vi "电流特性判定.vi"(7 "Result":refnum<vi>, 9 "索引":u8, 10 "判定参数":T1, 11 "XY曲线":cluster{"X":dbl[], "Y":dbl[]}[](array[cluster])) -> (2 "判定项长度":i32, 3 "OK？":bool)   [LabVIEW 2020]
panel:
  out "对称性检测点":dbl
  out "目标5逆向输入扭矩":dbl
  out "目标5正向输入扭矩":dbl
  out "目标 5":dbl
  out "目标4逆向输入扭矩":dbl
  out "目标4正向输入扭矩":dbl
  out "目标 4":dbl
  out "目标3逆向输入扭矩":dbl
  out "目标3正向输入扭矩":dbl
  out "目标 3":dbl
  out "目标2逆向输入扭矩":dbl
  out "目标2正向输入扭矩":dbl
  out "目标 2":dbl
  out "目标1正向输入扭矩":dbl
  out "目标1逆向输入扭矩":dbl
  out "目标 1":dbl
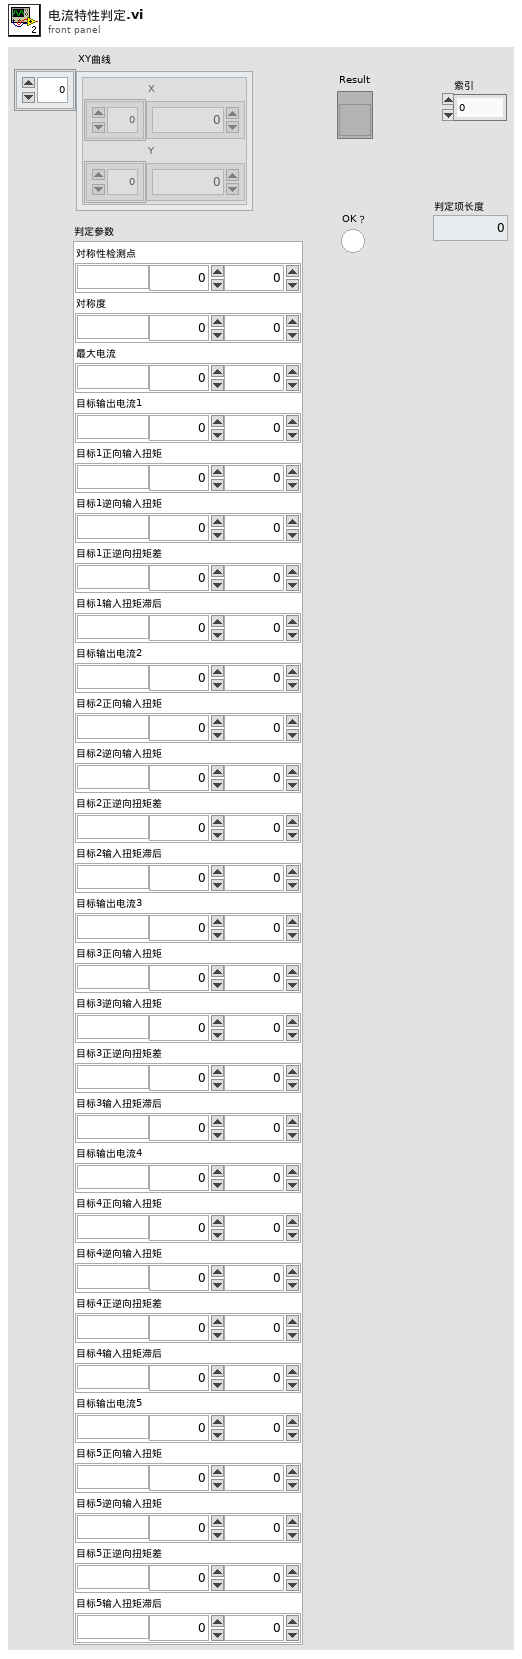
[diagram p1: front panel]
types:
  T1 = cluster{"对称性检测点":cluster{"单位":string, "下限":dbl, "上限":dbl}, "对称度":cluster{"单位":string, "下限":dbl, "上限":dbl}, "最大电流":cluster{"单位":string, "下限":dbl, "上限":dbl}, "目标输出电流1":cluster{"单位":string, "下限":dbl, "上限":dbl}, "目标1正向输入扭矩":cluster{"单位":string, "下限":dbl, "上限":dbl}, "目标1逆向输入扭矩":cluster{"单位":string, "下限":dbl, "上限":dbl}, "目标1正逆向扭矩差":cluster{"单位":string, "下限":dbl, "上限":dbl}, "目标1输入扭矩滞后":cluster{"单位":string, "下限":dbl, "上限":dbl}, "目标输出电流2":cluster{"单位":string, "下限":dbl, "上限":dbl}, "目标2正向输入扭矩":cluster{"单位":string, "下限":dbl, "上限":dbl}, "目标2逆向输入扭矩":cluster{"单位":string, "下限":dbl, "上限":dbl}, "目标2正逆向扭矩差":cluster{"单位":string, "下限":dbl, "上限":dbl}, "目标2输入扭矩滞后":cluster{"单位":string, "下限":dbl, "上限":dbl}, "目标输出电流3":cluster{"单位":string, "下限":dbl, "上限":dbl}, "目标3正向输入扭矩":cluster{"单位":string, "下限":dbl, "上限":dbl}, "目标3逆向输入扭矩":cluster{"单位":string, "下限":dbl, "上限":dbl}, "目标3正逆向扭矩差":cluster{"单位":string, "下限":dbl, "上限":dbl}, "目标3输入扭矩滞后":cluster{"单位":string, "下限":dbl, "上限":dbl}, "目标输出电流4":cluster{"单位":string, "下限":dbl, "上限":dbl}, "目标4正向输入扭矩":cluster{"单位":string, "下限":dbl, "上限":dbl}, "目标4逆向输入扭矩":cluster{"单位":string, "下限":dbl, "上限":dbl}, "目标4正逆向扭矩差":cluster{"单位":string, "下限":dbl, "上限":dbl}, "目标4输入扭矩滞后":cluster{"单位":string, "下限":dbl, "上限":dbl}, "目标输出电流5":cluster{"单位":string, "下限":dbl, "上限":dbl}, "目标5正向输入扭矩":cluster{"单位":string, "下限":dbl, "上限":dbl}, "目标5逆向输入扭矩":cluster{"单位":string, "下限":dbl, "上限":dbl}, "目标5正逆向扭矩差":cluster{"单位":string, "下限":dbl, "上限":dbl}, "目标5输入扭矩滞后":cluster{"单位":string, "下限":dbl, "上限":dbl}}
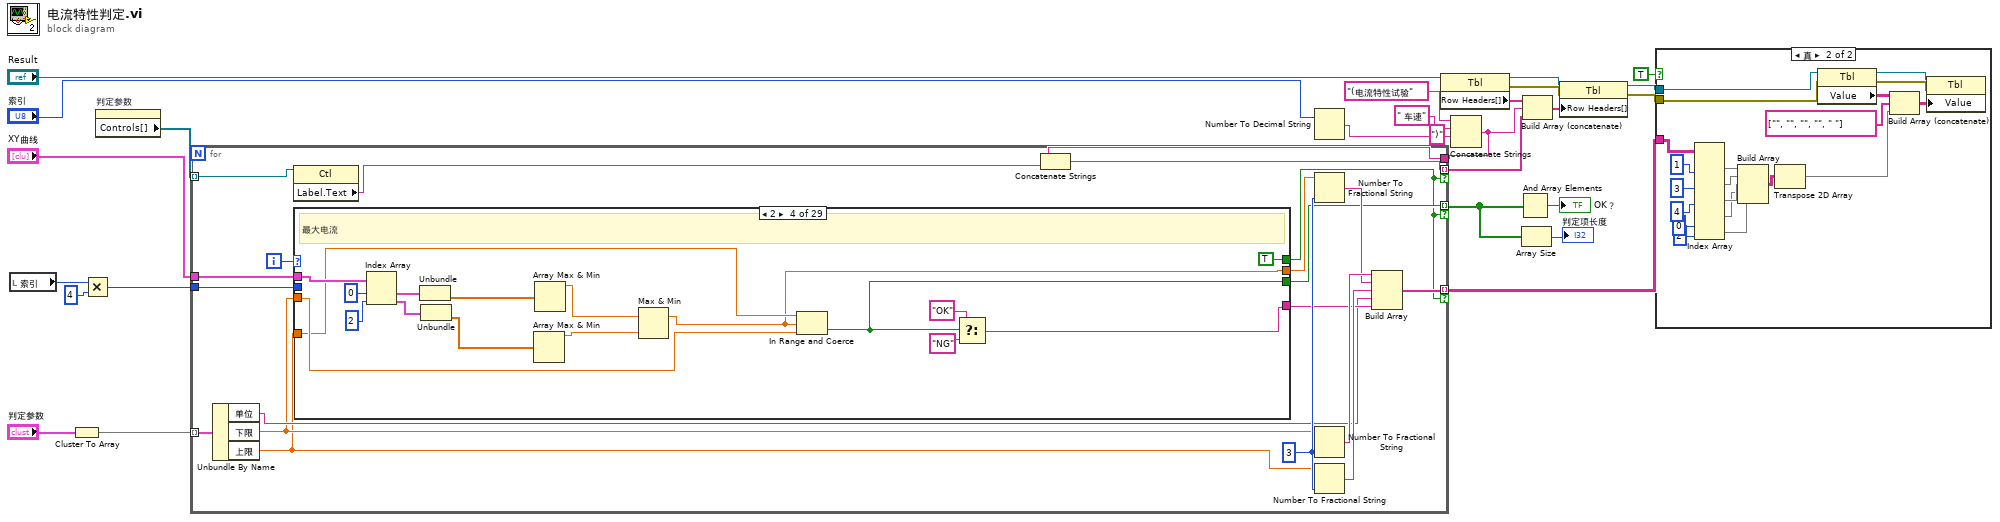
[diagram p0: block diagram]
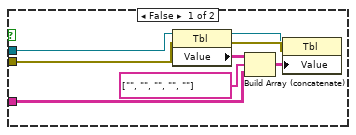
[diagram p2: hidden frame]
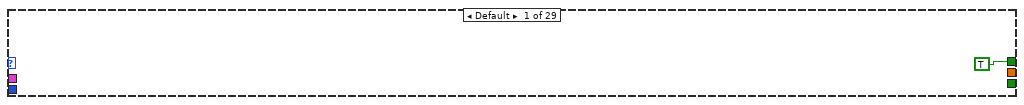
[diagram p3: hidden frame]
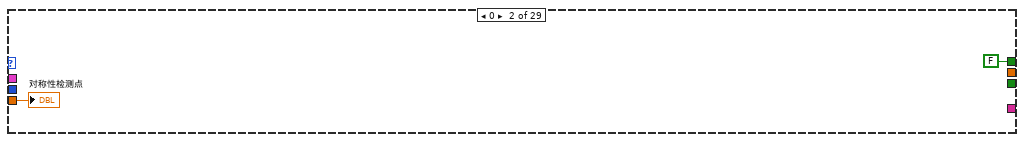
[diagram p4: hidden frame]
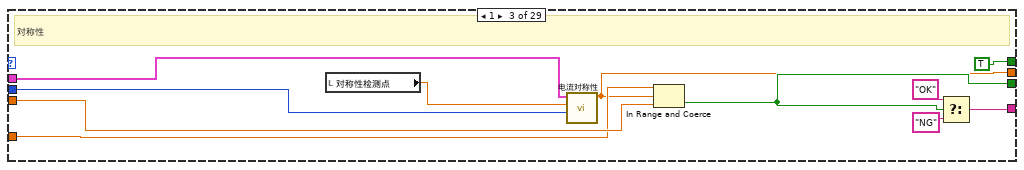
[diagram p5: hidden frame]
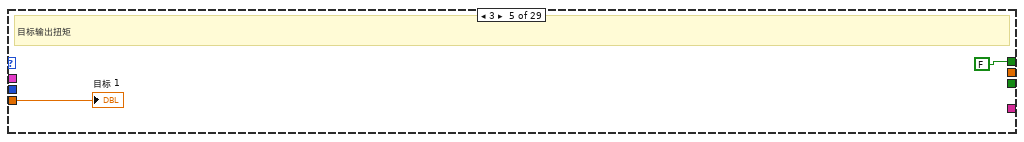
[diagram p6: hidden frame]
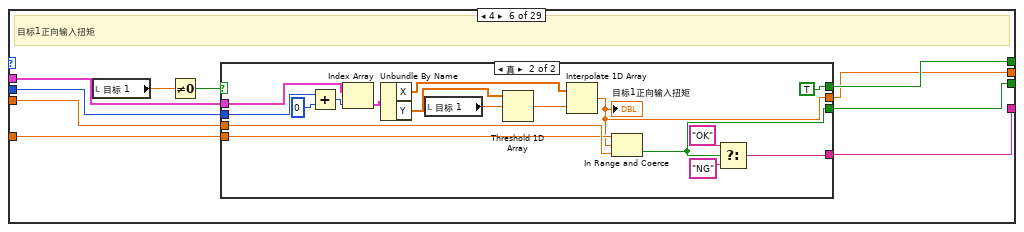
[diagram p7: hidden frame]
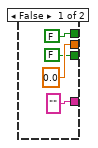
[diagram p8: hidden frame]
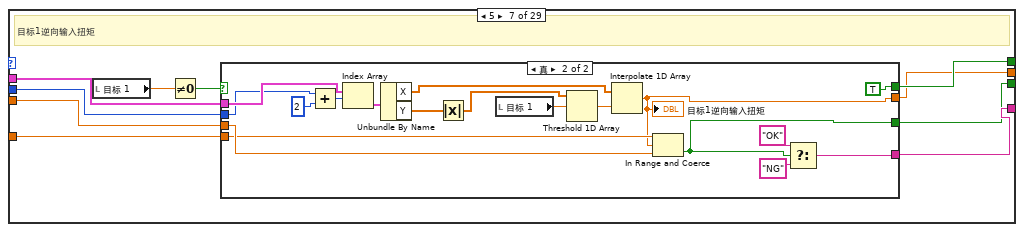
[diagram p9: hidden frame]
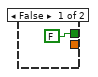
[diagram p10: hidden frame]
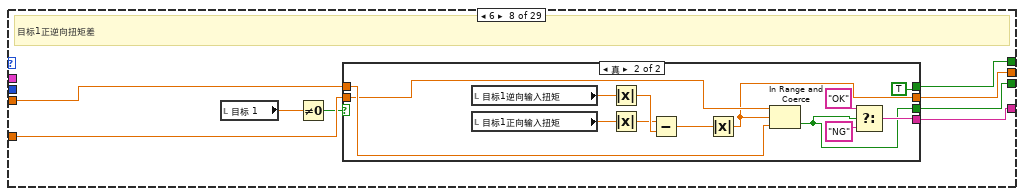
[diagram p11: hidden frame]
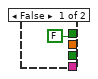
[diagram p12: hidden frame]
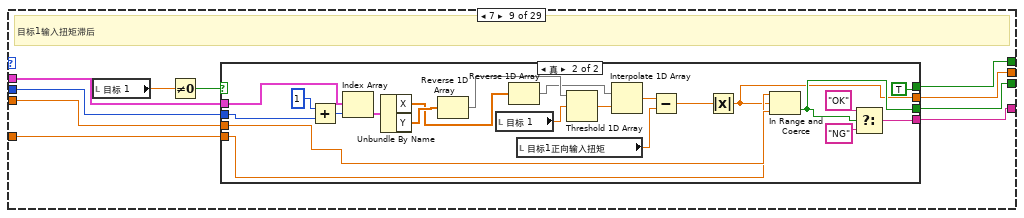
[diagram p13: hidden frame]
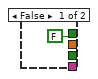
[diagram p14: hidden frame]
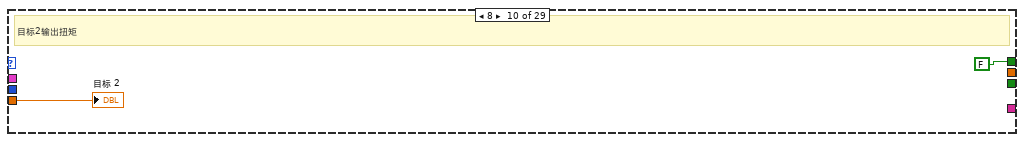
[diagram p15: hidden frame]
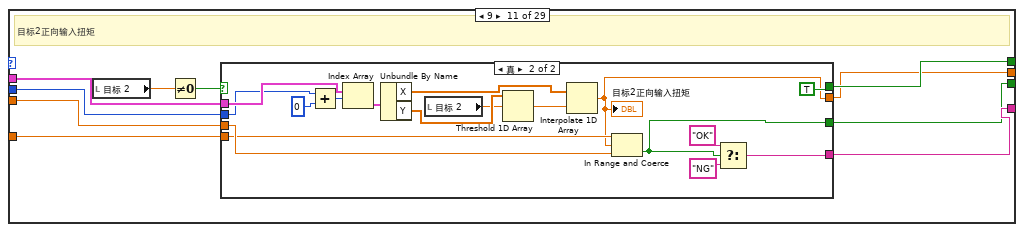
[diagram p16: hidden frame]
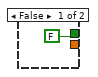
[diagram p17: hidden frame]
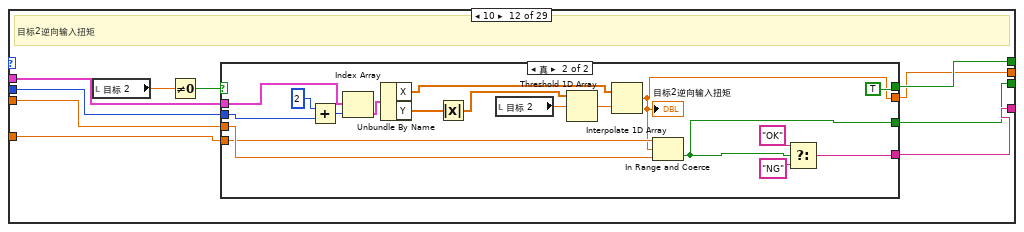
[diagram p18: hidden frame]
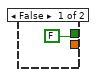
[diagram p19: hidden frame]
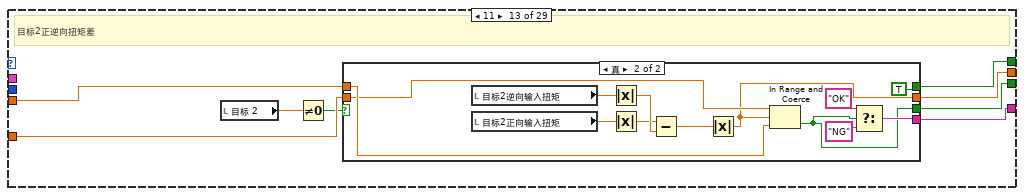
[diagram p20: hidden frame]
diagram:
  n1 = local read "索引"() -> (w7:u8)
  n2 = Cluster To Array(cluster="判定参数") -> (array=w26:cluster{"单位":string, "下限":dbl, "上限":dbl}[])
  n3 = Multiply(x=w7, y=u8 4) -> (x*y=w5:u8)
  n4 = property on="判定参数" class="Clust (严格)"() -> ("Controls[]"=w13:refnum<vi>[])  [unwired: 2 in, 2 out]
  n5 = Number To Decimal String(number="索引") -> (decimal integer string=w10:string)  [unwired: 1 in]
  n6 = property class="Tbl"(reference="Result") -> (reference out=w20:refnum<vi>, error out=w23:errorcluster, "Row Headers[]"=w16:string[])  [unwired: 1 in]
  n7 = Concatenate Strings("(电流特性试验" ("Label.Text"), " 车速" ("字符串"), w10, ")" ("字符串")) -> (w1:string)
  n8 = for {
    tunnel: w26 -> [w46] mode=indexing
    tunnel: w13 -> [w44] mode=indexing
    tunnel: "XY曲线" -> [w42]
    tunnel: [w36] -> w4 mode=indexing if=w30
    tunnel: [w32] -> w15 mode=indexing if=w30
    tunnel: [w28] -> w18 mode=indexing if=w30
    tunnel: w5 -> [w29]
    tunnel: w1 -> [w27]
    i -> [w45]
    w41 = i16 3 ("精度(6)")
    n9 = Unbundle By Name(w46) -> ("单位"=w35:string, "下限"=w34:dbl, "上限"=w33:dbl)
    n10 = property class="Ctl"(reference=w44) -> ("Label.Text"=w31:string)  [unwired: 1 in, 2 out]
    n11 = case shown="2" w45 {
      tunnel: [_ _ w52 w62 _ w83 w114 w142 w166 _ w200 w228 w256 w280 _ w314 w342 w370 w394 _ w428 w456 w484 w508 _ w542 w570 w598 w622] -> w43
      tunnel: w42 -> [_ _ w53 w76 _ w84 w115 _ w171 _ w201 w229 _ w285 _ w315 w343 _ w399 _ w429 w457 _ w513 _ w543 w571 _ w627]
      tunnel: [_ _ w58 w61 _ w89 w120 w147 w167 _ w206 w234 w261 w281 _ w320 w348 w375 w395 _ w434 w462 w489 w509 _ w548 w576 w603 w623] -> w37
      tunnel: [_ _ w57 w63 _ w88 w119 w146 w168 _ w205 w233 w260 w282 _ w319 w347 w374 w396 _ w433 w461 w488 w510 _ w547 w575 w602 w624] -> w36
      tunnel: w34 -> [_ w49 w56 w65 w78 w87 w118 w145 w170 w195 w204 w232 w259 w284 w309 w318 w346 w373 w398 w423 w432 w460 w487 w512 w537 w546 w574 w601 w626]
      tunnel: w33 -> [_ _ w55 w64 _ w86 w117 w144 w169 _ w203 w231 w258 w283 _ w317 w345 w372 w397 _ w431 w459 w486 w511 _ w545 w573 w600 w625]
      tunnel: [TRUE FALSE TRUE TRUE FALSE w85 w116 w143 w165 FALSE w202 w230 w257 w279 FALSE w316 w344 w371 w393 FALSE w430 w458 w485 w507 FALSE w544 w572 w599 w621] -> w30
      tunnel: w29 -> [_ _ w51 _ _ w82 w113 _ w164 _ w199 w227 _ w278 _ w313 w341 _ w392 _ w427 w455 _ w506 _ w541 w569 _ w620]
      frame Default {
      }
      frame 0 {
        "对称性检测点" <- w49
      }
      frame 1 {
        # "对称性"
        n12 = local read "对称性检测点"() -> (w50:dbl)
        n13 = call "电流对称性.vi"("索引"=w51, "定点"=w50, "XY图"=w53) -> ("对称性"=w52:dbl)  [unwired: 8 in]
        n14 = In Range and Coerce(upper limit=w55, x=w52, lower limit=w56) -> (In Range?=w57:bool)  [unwired: 1 out]
        n15 = Select(t="OK", s=w57, f="NG") -> (s? t:f=w58:string)
      }
      frame 2 {
        # "最大电流"
        n16 = Index Array(array=w76, index #1=0 ("索引"), index #2=2 ("索引")) -> (element #1=w73:cluster{"X":dbl[], "Y":dbl[]}, element #2=w72:cluster{"X":dbl[], "Y":dbl[]})
        n17 = Unbundle(w73) -> ("Y"=w71:dbl[])  [unwired: 1 out]
        n18 = Unbundle(w72) -> ("Y"=w70:dbl[])  [unwired: 1 out]
        n19 = Array Max & Min(array=w70) -> (max value=w68:dbl)  [unwired: 3 out]
        n20 = Array Max & Min(array=w71) -> (max value=w69:dbl)  [unwired: 3 out]
        n21 = Max & Min(x=w69, y=w68) -> (max(x,y)=w62:dbl)  [unwired: 1 out]
        n22 = In Range and Coerce(upper limit=w64, x=w62, lower limit=w65) -> (In Range?=w63:bool)  [unwired: 1 out]
        n23 = Select(t="OK", s=w63, f="NG") -> (s? t:f=w61:string)
      }
      frame 3 {
        # "目标输出扭矩"
        "目标 1" <- w78
      }
      frame 4 {
        # "目标1正向输入扭矩"
        n24 = local read "目标 1"() -> (w81:dbl)
        n25 = Not Equal To 0?(x=w81) -> (x != 0?=w80:bool)
        n26 = case shown="真" w80 {
          tunnel: ["" w108] -> w89
          tunnel: [FALSE w107] -> w88
          tunnel: w87 -> [_ w106]
          tunnel: w86 -> [_ w105]
          tunnel: [FALSE TRUE] -> w85
          tunnel: w84 -> [_ w103]
          tunnel: [0.0 w96] -> w83
          tunnel: w82 -> [_ w94]
          frame False {
          }
          frame True {
            n27 = Add(x=w94, y=0 ("索引")) -> (x+y=w95:i32)
            n28 = Index Array(array=w103, index=w95) -> (element=w102:cluster{"X":dbl[], "Y":dbl[]})
            n29 = Unbundle By Name(w102) -> ("X"=w99:dbl[], "Y"=w101:dbl[])
            n30 = local read "目标 1"() -> (w100:dbl)
            n31 = Threshold 1D Array(2:w100, 3:w101) -> (0:w98:dbl)  [unwired: 1 in]
            n32 = Interpolate 1D Array(1:w98, 2:w99) -> (0:w96:dbl)
            "目标1正向输入扭矩" <- w96
            n33 = In Range and Coerce(upper limit=w105, x=w96, lower limit=w106) -> (In Range?=w107:bool)  [unwired: 1 out]
            n34 = Select(t="OK", s=w107, f="NG") -> (s? t:f=w108:string)
          }
        }
      }
      frame 5 {
        # "目标1逆向输入扭矩"
        n35 = local read "目标 1"() -> (w112:dbl)
        n36 = Not Equal To 0?(x=w112) -> (x != 0?=w111:bool)
        n37 = case shown="真" w111 {
          tunnel: [_ w137] -> w120
          tunnel: [_ w136] -> w119
          tunnel: w118 -> [_ w135]
          tunnel: w117 -> [_ w134]
          tunnel: [FALSE TRUE] -> w116
          tunnel: w115 -> [_ w132]
          tunnel: [_ w126] -> w114
          tunnel: w113 -> [_ w122]
          frame False {
          }
          frame True {
            n38 = Add(x=w122, y=2 ("索引")) -> (x+y=w123:i32)
            n39 = Index Array(array=w132, index=w123) -> (element=w131:cluster{"X":dbl[], "Y":dbl[]})
            n40 = Unbundle By Name(w131) -> ("X"=w128:dbl[], "Y"=w130:dbl[])
            n41 = Absolute Value(x=w130) -> (abs(x)=w124:dbl[])
            n42 = local read "目标 1"() -> (w129:dbl)
            n43 = Threshold 1D Array(2:w129, 3:w124) -> (0:w127:dbl)  [unwired: 1 in]
            n44 = Interpolate 1D Array(1:w127, 2:w128) -> (0:w126:dbl)
            "目标1逆向输入扭矩" <- w126
            n45 = In Range and Coerce(upper limit=w134, x=w126, lower limit=w135) -> (In Range?=w136:bool)  [unwired: 1 out]
            n46 = Select(t="OK", s=w136, f="NG") -> (s? t:f=w137:string)
          }
        }
      }
      frame 6 {
        # "目标1正逆向扭矩差"
        n47 = local read "目标 1"() -> (w141:dbl)
        n48 = Not Equal To 0?(x=w141) -> (x != 0?=w140:bool)
        n49 = case shown="真" w140 {
          tunnel: [_ w159] -> w147
          tunnel: [_ w158] -> w146
          tunnel: w145 -> [_ w157]
          tunnel: w144 -> [_ w156]
          tunnel: [FALSE TRUE] -> w143
          tunnel: [_ w151] -> w142
          frame False {
          }
          frame True {
            n50 = local read "目标1逆向输入扭矩"() -> (w153:dbl)
            n51 = local read "目标1正向输入扭矩"() -> (w154:dbl)
            n52 = Absolute Value(x=w153) -> (abs(x)=w150:dbl)
            n53 = Absolute Value(x=w154) -> (abs(x)=w149:dbl)
            n54 = Subtract(x=w149, y=w150) -> (x-y=w152:dbl)
            n55 = Absolute Value(x=w152) -> (abs(x)=w151:dbl)
            n56 = In Range and Coerce(upper limit=w156, x=w151, lower limit=w157) -> (In Range?=w158:bool)  [unwired: 1 out]
            n57 = Select(t="OK", s=w158, f="NG") -> (s? t:f=w159:string)
          }
        }
      }
      frame 7 {
        # "目标1输入扭矩滞后"
        n58 = local read "目标 1"() -> (w163:dbl)
        n59 = Not Equal To 0?(x=w163) -> (x != 0?=w162:bool)
        n60 = case shown="真" w162 {
          tunnel: w171 -> [_ w188]
          tunnel: w170 -> [_ w182]
          tunnel: w169 -> [_ w181]
          tunnel: [_ w178] -> w168
          tunnel: [_ w177] -> w167
          tunnel: [_ w176] -> w166
          tunnel: [FALSE TRUE] -> w165
          tunnel: w164 -> [_ w173]
          frame False {
          }
          frame True {
            n61 = Add(x=1 ("索引"), y=w173) -> (x+y=w174:i32)
            n62 = Index Array(array=w188, index=w174) -> (element=w194:cluster{"X":dbl[], "Y":dbl[]})
            n63 = Unbundle By Name(w194) -> ("X"=w191:dbl[], "Y"=w193:dbl[])
            n64 = Reverse 1D Array(array=w193) -> (reversed array=w187:dbl[])
            n65 = local read "目标 1"() -> (w192:dbl)
            n66 = Reverse 1D Array(array=w191) -> (reversed array=w186:dbl[])
            n67 = local read "目标1正向输入扭矩"() -> (w184:dbl)
            n68 = Threshold 1D Array(2:w192, 3:w187) -> (0:w190:dbl)  [unwired: 1 in]
            n69 = Interpolate 1D Array(1:w190, 2:w186) -> (0:w185:dbl)
            n70 = Subtract(x=w185, y=w184) -> (x-y=w183:dbl)
            n71 = Absolute Value(x=w183) -> (abs(x)=w176:dbl)
            n72 = In Range and Coerce(upper limit=w181, x=w176, lower limit=w182) -> (In Range?=w178:bool)  [unwired: 1 out]
            n73 = Select(t="OK", s=w178, f="NG") -> (s? t:f=w177:string)
          }
        }
      }
      frame 8 {
        # "目标2输出扭矩"
        "目标 2" <- w195
      }
      frame 9 {
        # "目标2正向输入扭矩"
        n74 = local read "目标 2"() -> (w198:dbl)
        n75 = Not Equal To 0?(x=w198) -> (x != 0?=w197:bool)
        n76 = case shown="真" w197 {
          tunnel: [_ w222] -> w206
          tunnel: [_ w221] -> w205
          tunnel: w204 -> [_ w220]
          tunnel: w203 -> [_ w219]
          tunnel: [FALSE TRUE] -> w202
          tunnel: w201 -> [_ w217]
          tunnel: [_ w210] -> w200
          tunnel: w199 -> [_ w208]
          frame False {
          }
          frame True {
            n77 = Add(x=w208, y=0 ("索引")) -> (x+y=w209:i32)
            n78 = Index Array(array=w217, index=w209) -> (element=w216:cluster{"X":dbl[], "Y":dbl[]})
            n79 = Unbundle By Name(w216) -> ("X"=w213:dbl[], "Y"=w215:dbl[])
            n80 = local read "目标 2"() -> (w214:dbl)
            n81 = Threshold 1D Array(2:w214, 3:w215) -> (0:w212:dbl)  [unwired: 1 in]
            n82 = Interpolate 1D Array(1:w212, 2:w213) -> (0:w210:dbl)
            "目标2正向输入扭矩" <- w210
            n83 = In Range and Coerce(upper limit=w219, x=w210, lower limit=w220) -> (In Range?=w221:bool)  [unwired: 1 out]
            n84 = Select(t="OK", s=w221, f="NG") -> (s? t:f=w222:string)
          }
        }
      }
      frame 10 {
        # "目标2逆向输入扭矩"
        n85 = local read "目标 2"() -> (w226:dbl)
        n86 = Not Equal To 0?(x=w226) -> (x != 0?=w225:bool)
        n87 = case shown="真" w225 {
          tunnel: [_ w251] -> w234
          tunnel: [_ w250] -> w233
          tunnel: w232 -> [_ w249]
          tunnel: w231 -> [_ w248]
          tunnel: [FALSE TRUE] -> w230
          tunnel: w229 -> [_ w246]
          tunnel: [_ w240] -> w228
          tunnel: w227 -> [_ w236]
          frame False {
          }
          frame True {
            n88 = Add(x=2 ("索引"), y=w236) -> (x+y=w237:i32)
            n89 = Index Array(array=w246, index=w237) -> (element=w245:cluster{"X":dbl[], "Y":dbl[]})
            n90 = Unbundle By Name(w245) -> ("X"=w242:dbl[], "Y"=w244:dbl[])
            n91 = Absolute Value(x=w244) -> (abs(x)=w238:dbl[])
            n92 = local read "目标 2"() -> (w243:dbl)
            n93 = Threshold 1D Array(2:w243, 3:w238) -> (0:w241:dbl)  [unwired: 1 in]
            n94 = Interpolate 1D Array(1:w241, 2:w242) -> (0:w240:dbl)
            "目标2逆向输入扭矩" <- w240
            n95 = In Range and Coerce(upper limit=w248, x=w240, lower limit=w249) -> (In Range?=w250:bool)  [unwired: 1 out]
            n96 = Select(t="OK", s=w250, f="NG") -> (s? t:f=w251:string)
          }
        }
      }
      frame 11 {
        # "目标2正逆向扭矩差"
        n97 = local read "目标 2"() -> (w255:dbl)
        n98 = Not Equal To 0?(x=w255) -> (x != 0?=w254:bool)
        n99 = case shown="真" w254 {
          tunnel: [_ w273] -> w261
          tunnel: [_ w272] -> w260
          tunnel: w259 -> [_ w271]
          tunnel: w258 -> [_ w270]
          tunnel: [FALSE TRUE] -> w257
          tunnel: [_ w265] -> w256
          frame False {
          }
          frame True {
            n100 = local read "目标2逆向输入扭矩"() -> (w267:dbl)
            n101 = local read "目标2正向输入扭矩"() -> (w268:dbl)
            n102 = Absolute Value(x=w267) -> (abs(x)=w264:dbl)
            n103 = Absolute Value(x=w268) -> (abs(x)=w263:dbl)
            n104 = Subtract(x=w263, y=w264) -> (x-y=w266:dbl)
            n105 = Absolute Value(x=w266) -> (abs(x)=w265:dbl)
            n106 = In Range and Coerce(upper limit=w270, x=w265, lower limit=w271) -> (In Range?=w272:bool)  [unwired: 1 out]
            n107 = Select(t="OK", s=w272, f="NG") -> (s? t:f=w273:string)
          }
        }
      }
      frame 12 {
        # "目标2输入扭矩滞后"
        n108 = local read "目标 2"() -> (w277:dbl)
        n109 = Not Equal To 0?(x=w277) -> (x != 0?=w276:bool)
        n110 = case shown="真" w276 {
          tunnel: w285 -> [_ w302]
          tunnel: w284 -> [_ w296]
          tunnel: w283 -> [_ w295]
          tunnel: [_ w292] -> w282
          tunnel: [_ w291] -> w281
          tunnel: [_ w290] -> w280
          tunnel: [FALSE TRUE] -> w279
          tunnel: w278 -> [_ w287]
          frame False {
          }
          frame True {
            n111 = Add(x=1 ("索引"), y=w287) -> (x+y=w288:i32)
            n112 = Index Array(array=w302, index=w288) -> (element=w308:cluster{"X":dbl[], "Y":dbl[]})
            n113 = Unbundle By Name(w308) -> ("X"=w305:dbl[], "Y"=w307:dbl[])
            n114 = Reverse 1D Array(array=w307) -> (reversed array=w301:dbl[])
            n115 = local read "目标 2"() -> (w306:dbl)
            n116 = Reverse 1D Array(array=w305) -> (reversed array=w300:dbl[])
            n117 = local read "目标2正向输入扭矩"() -> (w298:dbl)
            n118 = Threshold 1D Array(2:w306, 3:w301) -> (0:w304:dbl)  [unwired: 1 in]
            n119 = Interpolate 1D Array(1:w304, 2:w300) -> (0:w299:dbl)
            n120 = Subtract(x=w299, y=w298) -> (x-y=w297:dbl)
            n121 = Absolute Value(x=w297) -> (abs(x)=w290:dbl)
            n122 = In Range and Coerce(upper limit=w295, x=w290, lower limit=w296) -> (In Range?=w292:bool)  [unwired: 1 out]
            n123 = Select(t="OK", s=w292, f="NG") -> (s? t:f=w291:string)
          }
        }
      }
      frame 13 {
        # "目标输出扭矩"
        "目标 3" <- w309
      }
      frame 14 {
        # "目标3正向输入扭矩"
        n124 = local read "目标 3"() -> (w312:dbl)
        n125 = Not Equal To 0?(x=w312) -> (x != 0?=w311:bool)
        n126 = case shown="真" w311 {
          tunnel: [_ w336] -> w320
          tunnel: [_ w335] -> w319
          tunnel: w318 -> [_ w334]
          tunnel: w317 -> [_ w333]
          tunnel: [FALSE TRUE] -> w316
          tunnel: w315 -> [_ w331]
          tunnel: [_ w324] -> w314
          tunnel: w313 -> [_ w322]
          frame False {
          }
          frame True {
            n127 = Add(x=w322, y=0 ("索引")) -> (x+y=w323:i32)
            n128 = Index Array(array=w331, index=w323) -> (element=w330:cluster{"X":dbl[], "Y":dbl[]})
            n129 = Unbundle By Name(w330) -> ("X"=w327:dbl[], "Y"=w329:dbl[])
            n130 = local read "目标 3"() -> (w328:dbl)
            n131 = Threshold 1D Array(2:w328, 3:w329) -> (0:w326:dbl)  [unwired: 1 in]
            n132 = Interpolate 1D Array(1:w326, 2:w327) -> (0:w324:dbl)
            "目标3正向输入扭矩" <- w324
            n133 = In Range and Coerce(upper limit=w333, x=w324, lower limit=w334) -> (In Range?=w335:bool)  [unwired: 1 out]
            n134 = Select(t="OK", s=w335, f="NG") -> (s? t:f=w336:string)
          }
        }
      }
      frame 15 {
        # "目标3逆向输入扭矩"
        n135 = local read "目标 3"() -> (w340:dbl)
        n136 = Not Equal To 0?(x=w340) -> (x != 0?=w339:bool)
        n137 = case shown="真" w339 {
          tunnel: [_ w365] -> w348
          tunnel: [_ w364] -> w347
          tunnel: w346 -> [_ w363]
          tunnel: w345 -> [_ w362]
          tunnel: [FALSE TRUE] -> w344
          tunnel: w343 -> [_ w360]
          tunnel: [_ w354] -> w342
          tunnel: w341 -> [_ w350]
          frame False {
          }
          frame True {
            n138 = Add(x=w350, y=2 ("索引")) -> (x+y=w351:i32)
            n139 = Index Array(array=w360, index=w351) -> (element=w359:cluster{"X":dbl[], "Y":dbl[]})
            n140 = Unbundle By Name(w359) -> ("X"=w356:dbl[], "Y"=w358:dbl[])
            n141 = Absolute Value(x=w358) -> (abs(x)=w352:dbl[])
            n142 = local read "目标 3"() -> (w357:dbl)
            n143 = Threshold 1D Array(2:w357, 3:w352) -> (0:w355:dbl)  [unwired: 1 in]
            n144 = Interpolate 1D Array(1:w355, 2:w356) -> (0:w354:dbl)
            "目标3逆向输入扭矩" <- w354
            n145 = In Range and Coerce(upper limit=w362, x=w354, lower limit=w363) -> (In Range?=w364:bool)  [unwired: 1 out]
            n146 = Select(t="OK", s=w364, f="NG") -> (s? t:f=w365:string)
          }
        }
      }
      frame 16 {
        # "目标3正逆向扭矩差"
        n147 = local read "目标 3"() -> (w369:dbl)
        n148 = Not Equal To 0?(x=w369) -> (x != 0?=w368:bool)
        n149 = case shown="真" w368 {
          tunnel: [_ w387] -> w375
          tunnel: [_ w386] -> w374
          tunnel: w373 -> [_ w385]
          tunnel: w372 -> [_ w384]
          tunnel: [FALSE TRUE] -> w371
          tunnel: [_ w379] -> w370
          frame False {
          }
          frame True {
            n150 = local read "目标3逆向输入扭矩"() -> (w381:dbl)
            n151 = local read "目标3正向输入扭矩"() -> (w382:dbl)
            n152 = Absolute Value(x=w381) -> (abs(x)=w378:dbl)
            n153 = Absolute Value(x=w382) -> (abs(x)=w377:dbl)
            n154 = Subtract(x=w377, y=w378) -> (x-y=w380:dbl)
            n155 = Absolute Value(x=w380) -> (abs(x)=w379:dbl)
            n156 = In Range and Coerce(upper limit=w384, x=w379, lower limit=w385) -> (In Range?=w386:bool)  [unwired: 1 out]
            n157 = Select(t="OK", s=w386, f="NG") -> (s? t:f=w387:string)
          }
        }
      }
      frame 17 {
        # "目标3输入扭矩滞后"
        n158 = local read "目标 3"() -> (w391:dbl)
        n159 = Not Equal To 0?(x=w391) -> (x != 0?=w390:bool)
        n160 = case shown="真" w390 {
          tunnel: w399 -> [_ w416]
          tunnel: w398 -> [_ w410]
          tunnel: w397 -> [_ w409]
          tunnel: [_ w406] -> w396
          tunnel: [_ w405] -> w395
          tunnel: [_ w404] -> w394
          tunnel: [FALSE TRUE] -> w393
          tunnel: w392 -> [_ w401]
          frame False {
          }
          frame True {
            n161 = Add(x=1 ("索引"), y=w401) -> (x+y=w402:i32)
            n162 = Index Array(array=w416, index=w402) -> (element=w422:cluster{"X":dbl[], "Y":dbl[]})
            n163 = Unbundle By Name(w422) -> ("X"=w419:dbl[], "Y"=w421:dbl[])
            n164 = Reverse 1D Array(array=w421) -> (reversed array=w415:dbl[])
            n165 = local read "目标 3"() -> (w420:dbl)
            n166 = Reverse 1D Array(array=w419) -> (reversed array=w414:dbl[])
            n167 = local read "目标3正向输入扭矩"() -> (w412:dbl)
            n168 = Threshold 1D Array(2:w420, 3:w415) -> (0:w418:dbl)  [unwired: 1 in]
            n169 = Interpolate 1D Array(1:w418, 2:w414) -> (0:w413:dbl)
            n170 = Subtract(x=w413, y=w412) -> (x-y=w411:dbl)
            n171 = Absolute Value(x=w411) -> (abs(x)=w404:dbl)
            n172 = In Range and Coerce(upper limit=w409, x=w404, lower limit=w410) -> (In Range?=w406:bool)  [unwired: 1 out]
            n173 = Select(t="OK", s=w406, f="NG") -> (s? t:f=w405:string)
          }
        }
      }
      frame 18 {
        # "目标4输出扭矩"
        "目标 4" <- w423
      }
      frame 19 {
        # "目标4正向输入扭矩"
        n174 = local read "目标 4"() -> (w426:dbl)
        n175 = Not Equal To 0?(x=w426) -> (x != 0?=w425:bool)
        n176 = case shown="真" w425 {
          tunnel: [_ w450] -> w434
          tunnel: [_ w449] -> w433
          tunnel: w432 -> [_ w448]
          tunnel: w431 -> [_ w447]
          tunnel: [FALSE TRUE] -> w430
          tunnel: w429 -> [_ w445]
          tunnel: [_ w438] -> w428
          tunnel: w427 -> [_ w436]
          frame False {
          }
          frame True {
            n177 = Add(x=w436, y=0 ("索引")) -> (x+y=w437:i32)
            n178 = Index Array(array=w445, index=w437) -> (element=w444:cluster{"X":dbl[], "Y":dbl[]})
            n179 = Unbundle By Name(w444) -> ("X"=w441:dbl[], "Y"=w443:dbl[])
            n180 = local read "目标 4"() -> (w442:dbl)
            n181 = Threshold 1D Array(2:w442, 3:w443) -> (0:w440:dbl)  [unwired: 1 in]
            n182 = Interpolate 1D Array(1:w440, 2:w441) -> (0:w438:dbl)
            "目标4正向输入扭矩" <- w438
            n183 = In Range and Coerce(upper limit=w447, x=w438, lower limit=w448) -> (In Range?=w449:bool)  [unwired: 1 out]
            n184 = Select(t="OK", s=w449, f="NG") -> (s? t:f=w450:string)
          }
        }
      }
      frame 20 {
        # "目标4逆向输入扭矩"
        n185 = local read "目标 4"() -> (w454:dbl)
        n186 = Not Equal To 0?(x=w454) -> (x != 0?=w453:bool)
        n187 = case shown="真" w453 {
          tunnel: [_ w479] -> w462
          tunnel: [_ w478] -> w461
          tunnel: w460 -> [_ w477]
          tunnel: w459 -> [_ w476]
          tunnel: [FALSE TRUE] -> w458
          tunnel: w457 -> [_ w474]
          tunnel: [_ w468] -> w456
          tunnel: w455 -> [_ w464]
          frame False {
          }
          frame True {
            n188 = Add(x=w464, y=2 ("索引")) -> (x+y=w465:i32)
            n189 = Index Array(array=w474, index=w465) -> (element=w473:cluster{"X":dbl[], "Y":dbl[]})
            n190 = Unbundle By Name(w473) -> ("X"=w470:dbl[], "Y"=w472:dbl[])
            n191 = Absolute Value(x=w472) -> (abs(x)=w466:dbl[])
            n192 = local read "目标 4"() -> (w471:dbl)
            n193 = Threshold 1D Array(2:w471, 3:w466) -> (0:w469:dbl)  [unwired: 1 in]
            n194 = Interpolate 1D Array(1:w469, 2:w470) -> (0:w468:dbl)
            "目标4逆向输入扭矩" <- w468
            n195 = In Range and Coerce(upper limit=w476, x=w468, lower limit=w477) -> (In Range?=w478:bool)  [unwired: 1 out]
            n196 = Select(t="OK", s=w478, f="NG") -> (s? t:f=w479:string)
          }
        }
      }
      frame 21 {
        # "目标4正逆向扭矩差"
        n197 = local read "目标 4"() -> (w483:dbl)
        n198 = Not Equal To 0?(x=w483) -> (x != 0?=w482:bool)
        n199 = case shown="真" w482 {
          tunnel: [_ w501] -> w489
          tunnel: [_ w500] -> w488
          tunnel: w487 -> [_ w499]
          tunnel: w486 -> [_ w498]
          tunnel: [FALSE TRUE] -> w485
          tunnel: [_ w493] -> w484
          frame False {
          }
          frame True {
            n200 = local read "目标4逆向输入扭矩"() -> (w495:dbl)
            n201 = local read "目标4正向输入扭矩"() -> (w496:dbl)
            n202 = Absolute Value(x=w495) -> (abs(x)=w492:dbl)
            n203 = Absolute Value(x=w496) -> (abs(x)=w491:dbl)
            n204 = Subtract(x=w491, y=w492) -> (x-y=w494:dbl)
            n205 = Absolute Value(x=w494) -> (abs(x)=w493:dbl)
            n206 = In Range and Coerce(upper limit=w498, x=w493, lower limit=w499) -> (In Range?=w500:bool)  [unwired: 1 out]
            n207 = Select(t="OK", s=w500, f="NG") -> (s? t:f=w501:string)
          }
        }
      }
      frame 22 {
        # "目标4输入扭矩滞后"
        n208 = local read "目标 4"() -> (w505:dbl)
        n209 = Not Equal To 0?(x=w505) -> (x != 0?=w504:bool)
        n210 = case shown="真" w504 {
          tunnel: w513 -> [_ w530]
          tunnel: w512 -> [_ w524]
          tunnel: w511 -> [_ w523]
          tunnel: [_ w520] -> w510
          tunnel: [_ w519] -> w509
          tunnel: [_ w518] -> w508
          tunnel: [FALSE TRUE] -> w507
          tunnel: w506 -> [_ w515]
          frame False {
          }
          frame True {
            n211 = Add(x=w515, y=1 ("索引")) -> (x+y=w516:i32)
            n212 = Index Array(array=w530, index=w516) -> (element=w536:cluster{"X":dbl[], "Y":dbl[]})
            n213 = Unbundle By Name(w536) -> ("X"=w533:dbl[], "Y"=w535:dbl[])
            n214 = Reverse 1D Array(array=w535) -> (reversed array=w529:dbl[])
            n215 = local read "目标 4"() -> (w534:dbl)
            n216 = Reverse 1D Array(array=w533) -> (reversed array=w528:dbl[])
            n217 = local read "目标4正向输入扭矩"() -> (w526:dbl)
            n218 = Threshold 1D Array(2:w534, 3:w529) -> (0:w532:dbl)  [unwired: 1 in]
            n219 = Interpolate 1D Array(1:w532, 2:w528) -> (0:w527:dbl)
            n220 = Subtract(x=w527, y=w526) -> (x-y=w525:dbl)
            n221 = Absolute Value(x=w525) -> (abs(x)=w518:dbl)
            n222 = In Range and Coerce(upper limit=w523, x=w518, lower limit=w524) -> (In Range?=w520:bool)  [unwired: 1 out]
            n223 = Select(t="OK", s=w520, f="NG") -> (s? t:f=w519:string)
          }
        }
      }
      frame 23 {
        # "目标5输出扭矩"
        "目标 5" <- w537
      }
      frame 24 {
        # "目标5正向输入扭矩"
        n224 = local read "目标 5"() -> (w540:dbl)
        n225 = Not Equal To 0?(x=w540) -> (x != 0?=w539:bool)
        n226 = case shown="真" w539 {
          tunnel: [_ w564] -> w548
          tunnel: [_ w563] -> w547
          tunnel: w546 -> [_ w562]
          tunnel: w545 -> [_ w561]
          tunnel: [FALSE TRUE] -> w544
          tunnel: w543 -> [_ w559]
          tunnel: [_ w552] -> w542
          tunnel: w541 -> [_ w550]
          frame False {
          }
          frame True {
            n227 = Add(x=0 ("索引"), y=w550) -> (x+y=w551:i32)
            n228 = Index Array(array=w559, index=w551) -> (element=w558:cluster{"X":dbl[], "Y":dbl[]})
            n229 = Unbundle By Name(w558) -> ("X"=w555:dbl[], "Y"=w557:dbl[])
            n230 = local read "目标 5"() -> (w556:dbl)
            n231 = Threshold 1D Array(2:w556, 3:w557) -> (0:w554:dbl)  [unwired: 1 in]
            n232 = Interpolate 1D Array(1:w554, 2:w555) -> (0:w552:dbl)
            "目标5正向输入扭矩" <- w552
            n233 = In Range and Coerce(upper limit=w561, x=w552, lower limit=w562) -> (In Range?=w563:bool)  [unwired: 1 out]
            n234 = Select(t="OK", s=w563, f="NG") -> (s? t:f=w564:string)
          }
        }
      }
      frame 25 {
        # "目标5逆向输入扭矩"
        n235 = local read "目标 5"() -> (w568:dbl)
        n236 = Not Equal To 0?(x=w568) -> (x != 0?=w567:bool)
        n237 = case shown="真" w567 {
          tunnel: [_ w593] -> w576
          tunnel: [_ w592] -> w575
          tunnel: w574 -> [_ w591]
          tunnel: w573 -> [_ w590]
          tunnel: [FALSE TRUE] -> w572
          tunnel: w571 -> [_ w588]
          tunnel: [_ w582] -> w570
          tunnel: w569 -> [_ w578]
          frame False {
          }
          frame True {
            n238 = Add(x=2 ("索引"), y=w578) -> (x+y=w579:i32)
            n239 = Index Array(array=w588, index=w579) -> (element=w587:cluster{"X":dbl[], "Y":dbl[]})
            n240 = Unbundle By Name(w587) -> ("X"=w584:dbl[], "Y"=w586:dbl[])
            n241 = Absolute Value(x=w586) -> (abs(x)=w580:dbl[])
            n242 = local read "目标 5"() -> (w585:dbl)
            n243 = Threshold 1D Array(2:w585, 3:w580) -> (0:w583:dbl)  [unwired: 1 in]
            n244 = Interpolate 1D Array(1:w583, 2:w584) -> (0:w582:dbl)
            "目标5逆向输入扭矩" <- w582
            n245 = In Range and Coerce(upper limit=w590, x=w582, lower limit=w591) -> (In Range?=w592:bool)  [unwired: 1 out]
            n246 = Select(t="OK", s=w592, f="NG") -> (s? t:f=w593:string)
          }
        }
      }
      frame 26 {
        # "目标5正逆向扭矩差"
        n247 = local read "目标 5"() -> (w597:dbl)
        n248 = Not Equal To 0?(x=w597) -> (x != 0?=w596:bool)
        n249 = case shown="真" w596 {
          tunnel: [_ w615] -> w603
          tunnel: [_ w614] -> w602
          tunnel: w601 -> [_ w613]
          tunnel: w600 -> [_ w612]
          tunnel: [FALSE TRUE] -> w599
          tunnel: [_ w607] -> w598
          frame False {
          }
          frame True {
            n250 = local read "目标5逆向输入扭矩"() -> (w609:dbl)
            n251 = local read "目标5正向输入扭矩"() -> (w610:dbl)
            n252 = Absolute Value(x=w609) -> (abs(x)=w606:dbl)
            n253 = Absolute Value(x=w610) -> (abs(x)=w605:dbl)
            n254 = Subtract(x=w605, y=w606) -> (x-y=w608:dbl)
            n255 = Absolute Value(x=w608) -> (abs(x)=w607:dbl)
            n256 = In Range and Coerce(upper limit=w612, x=w607, lower limit=w613) -> (In Range?=w614:bool)  [unwired: 1 out]
            n257 = Select(t="OK", s=w614, f="NG") -> (s? t:f=w615:string)
          }
        }
      }
      frame 27 {
        # "目标5输入扭矩滞后"
        n258 = local read "目标 5"() -> (w619:dbl)
        n259 = Not Equal To 0?(x=w619) -> (x != 0?=w618:bool)
        n260 = case shown="真" w618 {
          tunnel: w627 -> [_ w644]
          tunnel: w626 -> [_ w638]
          tunnel: w625 -> [_ w637]
          tunnel: [_ w634] -> w624
          tunnel: [_ w633] -> w623
          tunnel: [_ w632] -> w622
          tunnel: [FALSE TRUE] -> w621
          tunnel: w620 -> [_ w629]
          frame False {
          }
          frame True {
            n261 = Add(x=1 ("索引"), y=w629) -> (x+y=w630:i32)
            n262 = Index Array(array=w644, index=w630) -> (element=w650:cluster{"X":dbl[], "Y":dbl[]})
            n263 = Unbundle By Name(w650) -> ("X"=w647:dbl[], "Y"=w649:dbl[])
            n264 = Reverse 1D Array(array=w649) -> (reversed array=w643:dbl[])
            n265 = local read "目标 5"() -> (w648:dbl)
            n266 = Reverse 1D Array(array=w647) -> (reversed array=w642:dbl[])
            n267 = local read "目标5正向输入扭矩"() -> (w640:dbl)
            n268 = Threshold 1D Array(2:w648, 3:w643) -> (0:w646:dbl)  [unwired: 1 in]
            n269 = Interpolate 1D Array(1:w646, 2:w642) -> (0:w641:dbl)
            n270 = Subtract(x=w641, y=w640) -> (x-y=w639:dbl)
            n271 = Absolute Value(x=w639) -> (abs(x)=w632:dbl)
            n272 = In Range and Coerce(upper limit=w637, x=w632, lower limit=w638) -> (In Range?=w634:bool)  [unwired: 1 out]
            n273 = Select(t="OK", s=w634, f="NG") -> (s? t:f=w633:string)
          }
        }
      }
    }
    n274 = Concatenate Strings(w27, w31) -> (w28:string)
    n275 = Number To Fractional String(number=w43, precision (6)=w41) -> (F-format string=w39:string)  [unwired: 2 in]
    n276 = Number To Fractional String(number=w34, precision (6)=w41) -> (F-format string=w40:string)  [unwired: 2 in]
    n277 = Number To Fractional String(number=w33, precision (6)=w41) -> (F-format string=w38:string)  [unwired: 2 in]
    n278 = Build Array(w40, w39, w38, w35, w37) -> (w32:string[])
  }
  n279 = And Array Elements(Boolean array=w4) -> (logical AND=→"OK？":bool)
  n280 = Array Size(array=w4) -> (size(s)=→"判定项长度":i32)
  n281 = Build Array (concatenate)(w16, w1, w18) -> (w19:string[])
  n282 = property class="Tbl"(reference=w20, error in=w23, "Row Headers[]"=w19) -> (reference out=w21:refnum<vi>, error out=w22:errorcluster)
  n283 = case shown="真" TRUE {
    tunnel: w22 -> [w656 w676]
    tunnel: w21 -> [w653 w673]
    tunnel: w15 -> [w652 w664]
    frame False {
      n284 = property class="Tbl"(reference=w653, error in=w656) -> (reference out=w654:refnum<vi>, error out=w655:errorcluster, "Value"=w657:string[][])
      n285 = Build Array (concatenate)(w657, string[] ["", "", "", "", ""], w652) -> (w658:string[][])
      n286 = property class="Tbl"(reference=w654, error in=w655, "Value"=w658) -> ()  [unwired: 2 out]
    }
    frame True {
      n287 = Index Array(array=w664, index (col) #1=1 ("禁用的索引 (列)"), index (col) #2=3 ("索引 (列)"), index (col) #3=4 ("索引 (列)"), index (col) #4=0 ("索引 (列)"), index (col) #5=2 ("索引 (列)")) -> (element #1=w668:string[], element #2=w667:string[], element #3=w666:string[], element #4=w660:string[], element #5=w659:string[])  [unwired: 5 in]
      n288 = Build Array(w668, w667, w666, w660, w659) -> (w665:string[][])
      n289 = Transpose 2D Array(2D array=w665) -> (transposed array=w663:string[][])
      n290 = property class="Tbl"(reference=w673, error in=w676) -> (reference out=w674:refnum<vi>, error out=w675:errorcluster, "Value"=w677:string[][])
      n291 = Build Array (concatenate)(w677, string[] ["", "", "", "", " "], w663) -> (w678:string[][])
      n292 = property class="Tbl"(reference=w674, error in=w675, "Value"=w678) -> ()  [unwired: 2 out]
    }
  }
